vi "Write PressureSensor.vi"(10 "PressureSensor":refnum<class "PressureSensor.lvclass">, 11 "Model in":refnum<class "Model.lvclass">) -> (3 "Model out":refnum<class "Model.lvclass">)   [LabVIEW 2015, in "Model.lvclass"]
uses:
  Model.lvclass
  PressureSensor/PressureSensor/PressureSensor.lvclass
  Model.lvclass/Model.ctl
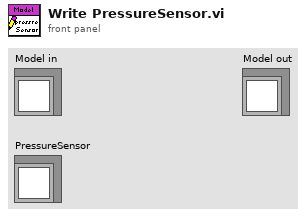
[diagram p1: front panel]
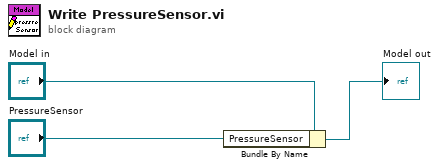
[diagram p0: block diagram]
diagram:
  n1 = Bundle By Name(cluster="Model in", "PressureSensor"="PressureSensor") -> (→"Model out":refnum<class "Model.lvclass">)
